vi "DAC_Write_OneChannel.vi"(8 "error in (no error)":errorcluster, 9 "Value":u16, 10 "Channel":u16, 11 "DeviceIndex":u64) -> (0 "error out":errorcluster, 3 "return type":u64)   [LabVIEW 2012]
uses:
  Windows/System32/AIOUSB.dll
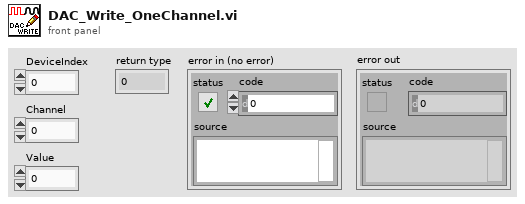
[diagram p1: front panel]
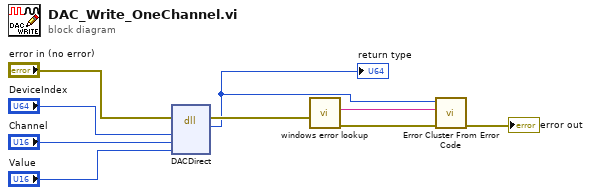
[diagram p0: block diagram]
diagram:
  n1 = dll-call lib="C:/Windows/System32/AIOUSB.dll" fn="DACDirect"(error in="error in (no error)", "DeviceIndex"="DeviceIndex", "Channel"="Channel", "Value"="Value") -> (error out=w2:errorcluster, "return type"=w1:u64)  [unwired: 5 in, 1 out]
  "return type" <- w1
  n2 = call "windows error lookup.vi"("error in (no error)"=w2) -> ("error out"=w4:errorcluster, "error message (\"\")"=w5:string)  [unwired: 9 in]
  n3 = call <vilib>:"Error Cluster From Error Code.vi"("error in (no error)"=w4, "error message (\"\")"=w5, "error code (0)"=w1) -> ("error out"=→"error out":errorcluster)  [unwired: 6 in]
